vi "Configure LO Sharing.vi"(0 "reference":refnum<k15>, 5 "Carrier Frequency [Hz]":dbl=5000000000.0 format="%#_6p", 7 "Gain":dbl=50.0, 11 "error in":errorcluster) -> (4 "reference out":refnum<k15>, 6 "Coerced Carrier Frequency":dbl format="%#_6p", 15 "error out":errorcluster)   [LabVIEW 2015]
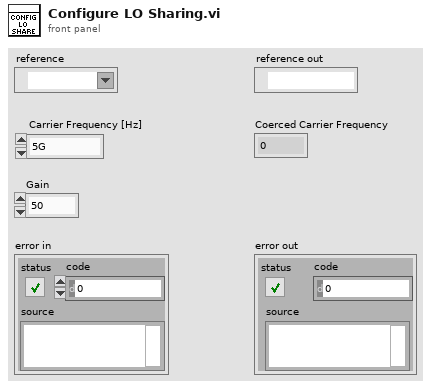
[diagram p1: front panel]
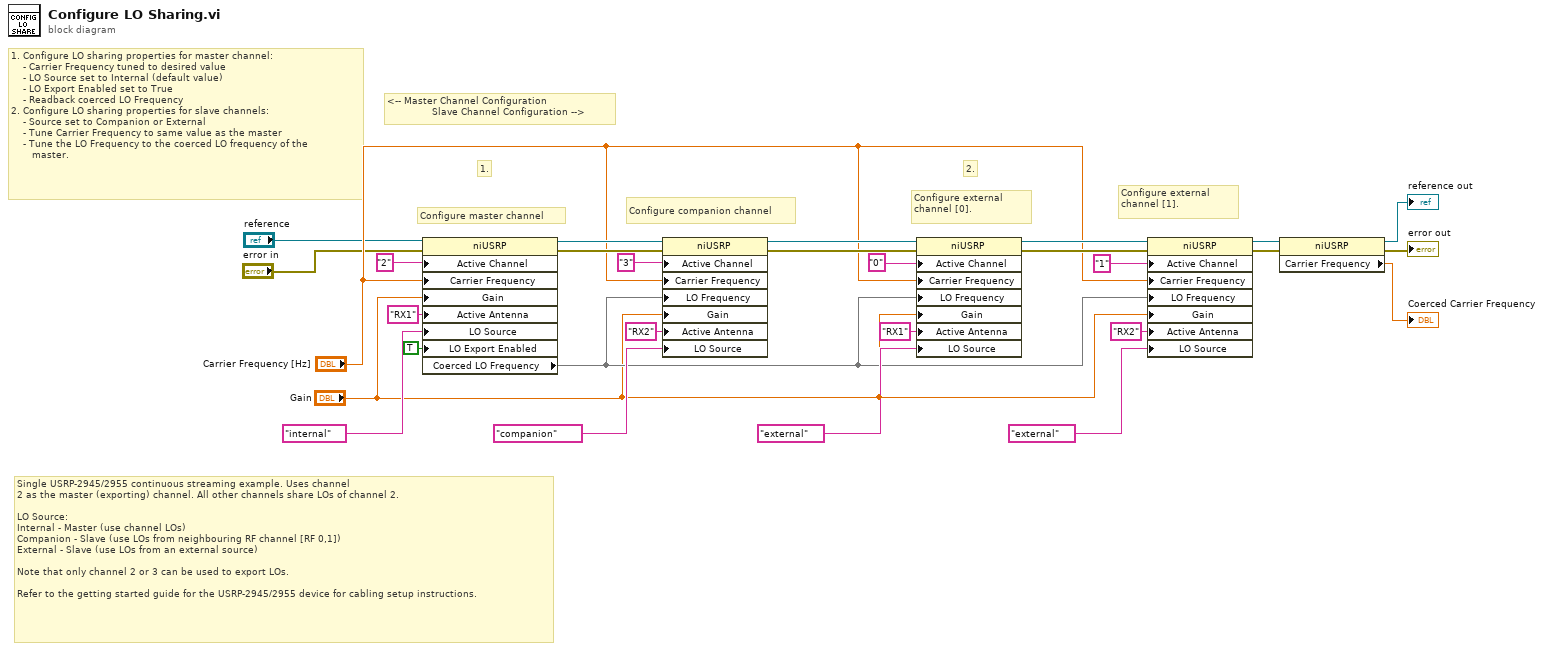
[diagram p0: block diagram]
diagram:
  # "2."
  # "1."
  # "1. Configure LO sharing properties for master channel:\n    - Carrier Frequency tuned to desired value\n    - LO Source set to Internal (default value)\n    - LO Export Enabled set to True\n    - Readback coerced LO Frequency\n2. Configure LO sharing properties for slave channels:\n    - Source set to Companion or External\n    - Tune Carrier Frequency to same value as the master\n    - Tune the LO Frequency to the coerced LO frequency of the \n       master."
  # "Single USRP-2945/2955 continuous streaming example. Uses channel\n2 as the master (exporting) channel. All other channels share LOs of channel 2.\n\nLO Source:\nInternal - Master (use channel LOs)\nCompanion - Slave (use LOs from neighbouring RF channel [RF 0,1])\nExternal - Slave (use LOs from an external source)\n\nNote that only channel 2 or 3 can be used to export LOs.\n\nRefer to the getting started guide for the USRP-2945/2955 device for cabling setup instructions."
  # "<-- Master Channel Configuration           \n               Slave Channel Configuration -->"
  # "Configure external channel [1]."
  # "Configure external channel [0]."
  # "Configure companion channel"
  # "Configure master channel"
  n1 = property class="niUSRP"(reference="reference", error in="error in", "Active Channel"="2", "Carrier Frequency"="Carrier Frequency [Hz]", "Gain"="Gain", "Active Antenna"="RX1" ("Configuration:Active Antenna"), "LO Source"="internal" ("Clocking and Synchronization:LO:LO Source"), "LO Export Enabled"=TRUE ("Clocking and Synchronization:LO:LO Export Enabled")) -> (reference out=w29:refnum<k15>, error out=w28:errorcluster, "Coerced LO Frequency"=w14)
  n2 = property class="niUSRP"(reference=w29, error in=w28, "Active Channel"="3", "Carrier Frequency"="Carrier Frequency [Hz]", "LO Frequency"=w14, "Gain"="Gain", "Active Antenna"="RX2" ("Configuration:Active Antenna"), "LO Source"="companion" ("Clocking and Synchronization:LO:LO Source")) -> (reference out=w25:refnum<k15>, error out=w23:errorcluster)
  n3 = property class="niUSRP"(reference=w25, error in=w23, "Active Channel"="0", "Carrier Frequency"="Carrier Frequency [Hz]", "LO Frequency"=w14, "Gain"="Gain", "Active Antenna"="RX1" ("Configuration:Active Antenna"), "LO Source"="external" ("Clocking and Synchronization:LO:LO Source")) -> (reference out=w16:refnum<k15>, error out=w24:errorcluster)
  n4 = property class="niUSRP"(reference=w16, error in=w24, "Active Channel"="1", "Carrier Frequency"="Carrier Frequency [Hz]", "LO Frequency"=w14, "Gain"="Gain", "Active Antenna"="RX2" ("Configuration:Active Antenna"), "LO Source"="external" ("Clocking and Synchronization:LO:LO Source")) -> (reference out=w3:refnum<k15>, error out=w5:errorcluster)
  n5 = property class="niUSRP"(reference=w3, error in=w5) -> (reference out=→"reference out":refnum<k15>, error out=→"error out":errorcluster, "Carrier Frequency"=→"Coerced Carrier Frequency":dbl)
